vi "FullMeasurementSubVI.vi"(0 "LINX Resource":T1, 1 "M0":bool, 2 "Stop REF":refnum<vi>, 3 "error in (no error)":errorcluster, 4 "M1":bool, 6 "Motor steps":i32) -> (5 "LINX Resource 2":T1, 7 "Array":dbl[](array[numeric]), 8 "error out":errorcluster)   [LabVIEW 2021]
uses:
  <vilib>/MakerHub/LINX/Private/Type Defs/LINX Ref.ctl
  <vilib>/MakerHub/LINX/Private/Type Defs/Platform.ctl
  <vilib>/MakerHub/LINX/Private/Type Defs/Interface.ctl
  <vilib>/MakerHub/LINX/Private/Device/Type Defs/LINX Device Config.ctl
  <vilib>/MakerHub/LINX/Private/Device/Type Defs/TCP Config.ctl
  <vilib>/MakerHub/LINX/Private/Device/Type Defs/Channels.ctl
  <vilib>/MakerHub/LINX/Public/Peripherals/Digital/Digital Write 1 Chan.vi
  <vilib>/MakerHub/LINX/Public/Peripherals/Digital/Digital Write N Chans.vi
  <vilib>/MakerHub/LINX/Private/Local IO/LinxDigitalWrite.vi
  <vilib>/MakerHub/LINX/Public/Utilities/Check Channel.vi
  <vilib>/MakerHub/LINX/Private/Utilties/Generate Error.vi
  <vilib>/MakerHub/LINX/LMH-LINX.lvlib
  <vilib>/MakerHub/LINX/Private/Device/Device.lvlib
panel:
  out "Adjusted motor steps":i32
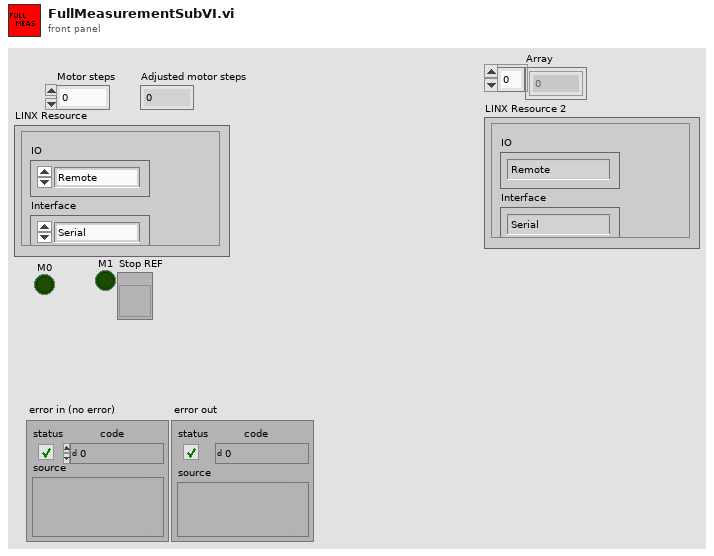
[diagram p1: front panel]
types:
  T1 = typedef "LMH-LINX.lvlib/LINX Ref.ctl" = cluster{"IO":T2, "Interface":T3, "LINX Device Config":T4}
  T2 = typedef "LMH-LINX.lvlib/Platform.ctl" = enum16{"Remote", "Local"}
  T3 = typedef "LMH-LINX.lvlib/Interface.ctl" = enum16{"Serial", "TCP"}
  T4 = typedef "LMH-LINX.lvlib/Device.lvlib/LINX Device Config.ctl" = cluster{"Interface":T3, "COM Port":refnum<visa-resource-name>, "TCP Configuration":T5, "Device Family":u8, "Device ID":u8, "Device Name":string, "TCP Ref":refnum<k5>, "Channels":T6}
  T5 = typedef "LMH-LINX.lvlib/Device.lvlib/TCP Config.ctl" = cluster{"IP Address":string, "Port":u16}
  T6 = typedef "LMH-LINX.lvlib/Channels.ctl" = cluster{"DI":u8[], "DO":u8[], "AI":u8[], "AO":u8[], "PWM":u8[], "QE":u8[], "UART":u8[], "I2C 2":u8[], "SPI":u8[], "CAN":u8[], "Servo":u8[], "AI Ref (V)":dbl, "AI Resolution (Bits)":u8, "AO Ref (V)":dbl, "AO Resolution (Bits)":u8}
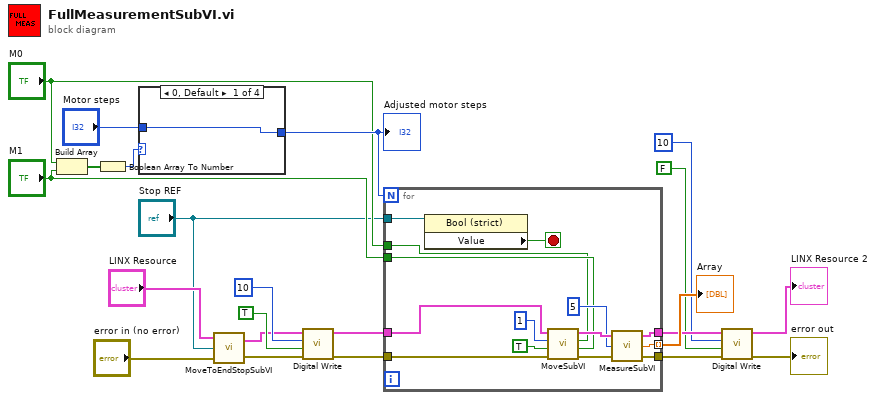
[diagram p0: block diagram]
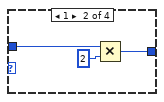
[diagram p2: hidden frame]
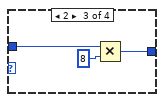
[diagram p3: hidden frame]
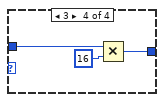
[diagram p4: hidden frame]
diagram:
  n1 = Build Array("M0", "M1") -> (w13:bool[])
  n2 = Boolean Array To Number(Boolean array=w13) -> (number=w12:u32)
  n3 = case shown="0, Default" w12 {
    tunnel: "Motor steps" -> [w23 w26 w28 w32]
    tunnel: [w23 w25 w29 w31] -> w10
    frame 0, Default {
    }
    frame 1 {
      n4 = Multiply(x=w26, y=2) -> (x*y=w25:i32)
    }
    frame 2 {
      n5 = Multiply(x=w28, y=8) -> (x*y=w29:i32)
    }
    frame 3 {
      n6 = Multiply(x=w32, y=16) -> (x*y=w31:i32)
    }
  }
  "Adjusted motor steps" <- w10
  n7 = call "MoveToEndStopSubVI.vi"("error in (no error)"="error in (no error)", "Boolean 2"="Stop REF", "LINX Resource"="LINX Resource") -> ("error out"=w1:errorcluster, "LINX Resource 2"=w2:T1)
  n8 = call-poly <vilib>:"Digital Write.vi"("Error In"=w1, "Output Value"=TRUE, "DO Channel"=u8 10, "LINX Resource"=w2) -> ("Error Out"=w18:errorcluster, "LINX Resource"=w21:T1)  [unwired: 6 in]
  n9 = for {
    N: w10 -> [_]
    tunnel: [w41] -> w22 mode=indexing
    tunnel: [w40] -> w20
    tunnel: [w39] -> w19
    tunnel: w21 -> [w38]
    tunnel: w18 -> [w37]
    tunnel: "M1" -> [w36]
    tunnel: "M0" -> [w35]
    tunnel: "Stop REF" -> [w33]
    stop <- w34 stop-if-true
    n10 = property class="Bool (strict)"(reference=w33) -> ("Value"=w34:bool)  [unwired: 1 in, 2 out]
    n11 = call "MoveSubVI.vi"("M1"=w36, "M0"=w35, "error in (no error)"=w37, "Direction"=TRUE, "Number of Steps"=u32 1, "LINX Resource"=w38) -> ("error out"=w45:errorcluster, "LINX Resource 2"=w46:T1)
    n12 = call "MeasureSubVI.vi"("error in (no error)"=w45, "Number of Samples"=5, "LINX Resource"=w46) -> ("error out"=w39:errorcluster, "Average"=w41:dbl, "LINX Resource 2"=w40:T1)
  }
  "Array" <- w22
  n13 = call-poly <vilib>:"Digital Write.vi"("Error In"=w19, "Output Value"=FALSE, "DO Channel"=u8 10, "LINX Resource"=w20) -> ("Error Out"=→"error out":errorcluster, "LINX Resource"=→"LINX Resource 2":T1)  [unwired: 6 in]
